vi "ReportVelocityState.vi"(1 "Destination":T3={"Subsystem Id"=90, "Node Id"=1, "Component Id"=1}, 2 "PresenceVector":u16=2 format="%b", 3 "VelocityState":T1, 4 "Source":T3={"Subsystem Id"=3, "Node Id"=1, "Component Id"=1}) -> (0 "Encoded JAUS Message":string)   [LabVIEW 2009]
uses:
  Support Files/Address.ctl
  Support Files/VelocityState.ctl
  Support Files/TimeRec.ctl
panel:
  in  "Command Code":string="D\u0004"
  # "Only Velocity X, Yaw Rate and Time Stamp need to be supplied"
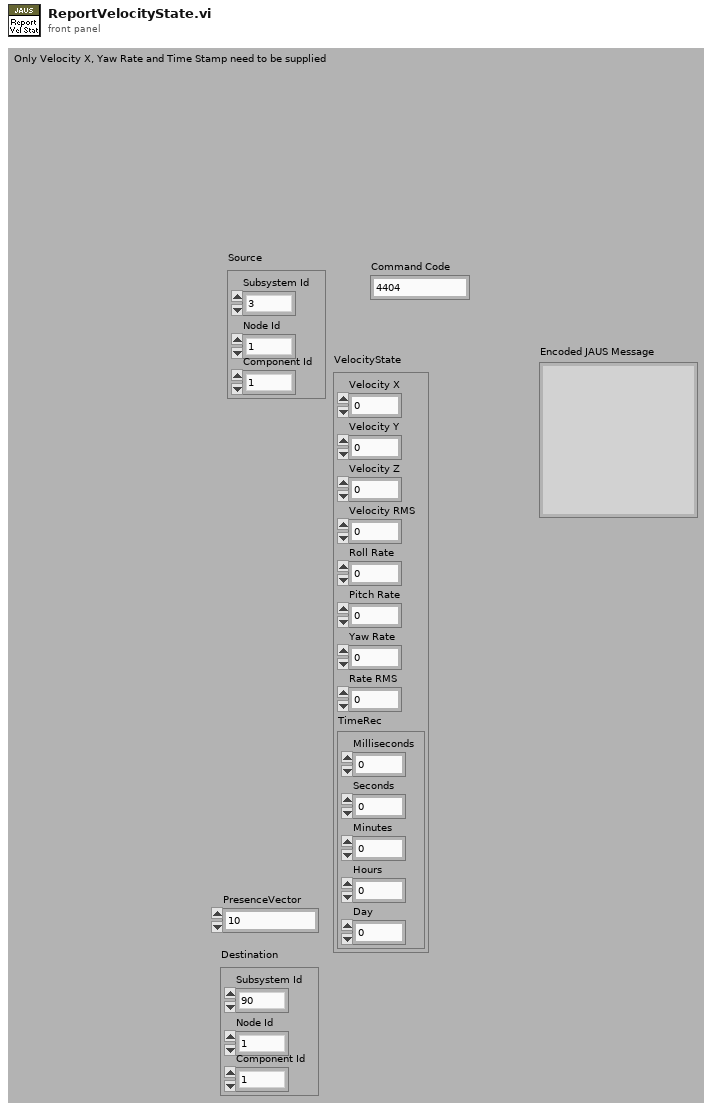
[diagram p1: front panel]
types:
  T1 = typedef "VelocityState.ctl" = cluster{"Velocity X":dbl, "Velocity Y":dbl, "Velocity Z":dbl, "Velocity RMS":dbl, "Roll Rate":dbl, "Pitch Rate":dbl, "Yaw Rate":dbl, "Rate RMS":dbl, "TimeRec":T2}
  T2 = typedef "TimeRec.ctl" = cluster{"Milliseconds":u32, "Seconds":u32, "Minutes":u32, "Hours":u32, "Day":u32}
  T3 = typedef "Address.ctl" = cluster{"Subsystem Id":u16, "Node Id":u8, "Component Id":u8}
  T4 = cluster{"unsigned byte array[0]":u8, "unsigned byte array[1]":u8}
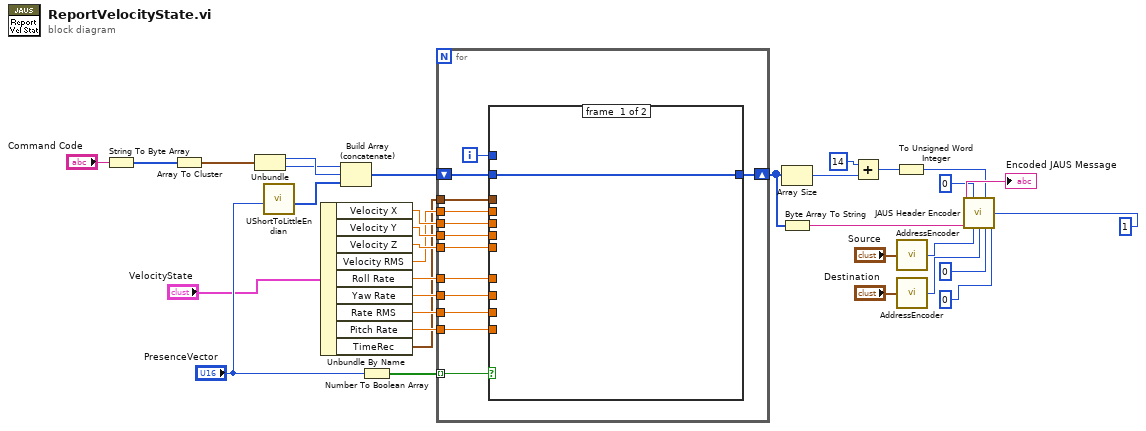
[diagram p0: block diagram]
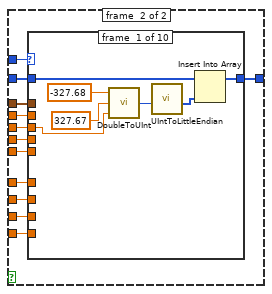
[diagram p2: hidden frame]
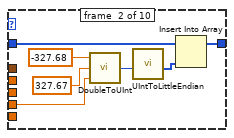
[diagram p3: hidden frame]
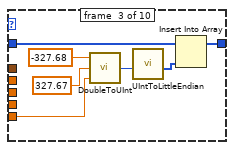
[diagram p4: hidden frame]
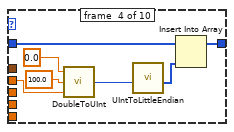
[diagram p5: hidden frame]
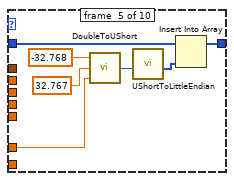
[diagram p6: hidden frame]
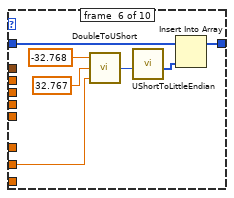
[diagram p7: hidden frame]
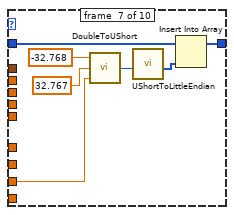
[diagram p8: hidden frame]
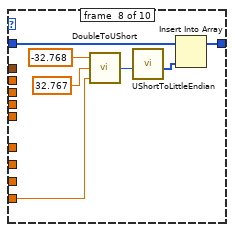
[diagram p9: hidden frame]
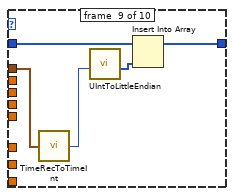
[diagram p10: hidden frame]
diagram:
  n1 = String To Byte Array(string="Command Code") -> (unsigned byte array=w17:u8[])
  n2 = Array To Cluster(array=w17) -> (cluster=w16:T4)
  n3 = Unbundle(w16) -> ("unsigned byte array[0]"=w15:u8, "unsigned byte array[1]"=w14:u8)
  n4 = call "UShortToLittleEndian.vi"("Number"="PresenceVector") -> ("byte array"=w22:u8[])  [unwired: 10 in]
  n5 = Unbundle By Name("VelocityState") -> ("Velocity X"=w13:dbl, "Velocity Y"=w12:dbl, "Velocity Z"=w11:dbl, "Velocity RMS"=w10:dbl, "Roll Rate"=w9:dbl, "Yaw Rate"=w8:dbl, "Rate RMS"=w7:dbl, "Pitch Rate"=w6:dbl, "TimeRec"=w5:T2)
  n6 = Build Array (concatenate)(w14, w15, w22) -> (w20:u8[])
  n7 = Number To Boolean Array(number="PresenceVector") -> (Boolean array=w25:bool[])
  n8 = for {
    tunnel: w25 -> [w47] mode=indexing
    tunnel: w13 -> [w45]
    tunnel: w12 -> [w44]
    tunnel: w11 -> [w43]
    tunnel: w10 -> [w42]
    tunnel: w9 -> [w41]
    tunnel: w8 -> [w40]
    tunnel: w7 -> [w39]
    tunnel: w6 -> [w38]
    tunnel: w5 -> [w37]
    shift-right: [w35] -> w19
    shift-left: w20 -> [w36]
    i -> [w46]
    n9 = case shown="True" w47 {
      tunnel: w46 -> [_ w60]
      tunnel: w45 -> [_ w59]
      tunnel: w44 -> [_ w58]
      tunnel: w43 -> [_ w57]
      tunnel: w42 -> [_ w56]
      tunnel: w41 -> [_ w55]
      tunnel: w40 -> [_ w54]
      tunnel: w39 -> [_ w53]
      tunnel: w38 -> [_ w52]
      tunnel: w37 -> [_ w51]
      tunnel: w36 -> [w48 w50]
      tunnel: [w48 w49] -> w35
      frame #0 {
      }
      frame #1 {
        n10 = case shown="8" w60 {
          tunnel: w59 -> [w63 _ _ _ _ _ _ _ _ _]
          tunnel: w58 -> [_ w70 _ _ _ _ _ _ _ _]
          tunnel: w57 -> [_ _ w77 _ _ _ _ _ _ _]
          tunnel: w56 -> [_ _ _ w84 _ _ _ _ _ _]
          tunnel: w55 -> [_ _ _ _ w91 _ _ _ _ _]
          tunnel: w54 -> [_ _ _ _ _ w98 _ _ _ _]
          tunnel: w53 -> [_ _ _ _ _ _ w105 _ _ _]
          tunnel: w52 -> [_ _ _ _ _ _ _ w112 _ _]
          tunnel: w51 -> [_ _ _ _ _ _ _ _ w120 _]
          tunnel: w50 -> [w62 w69 w76 w83 w90 w97 w104 w111 w118 w122]
          tunnel: [w61 w68 w75 w82 w89 w96 w103 w110 w117 w122] -> w49
          frame #0 {
            n11 = call "DoubleToUInt.vi"("Value"=w63, "Max"=327.67, "Min"=-327.68) -> ("scaled Integer"=w65:u32)
            n12 = call "UIntToLittleEndian.vi"("Number"=w65) -> ("byte array"=w64:u8[])  [unwired: 10 in]
            n13 = Insert Into Array(array=w62, new element=w64) -> (w61:u8[])  [unwired: 1 in]
          }
          frame #1 {
            n14 = call "DoubleToUInt.vi"("Value"=w70, "Max"=327.67, "Min"=-327.68) -> ("scaled Integer"=w72:u32)
            n15 = call "UIntToLittleEndian.vi"("Number"=w72) -> ("byte array"=w71:u8[])  [unwired: 10 in]
            n16 = Insert Into Array(array=w69, new element=w71) -> (w68:u8[])  [unwired: 1 in]
          }
          frame #2 {
            n17 = call "DoubleToUInt.vi"("Value"=w77, "Max"=327.67, "Min"=-327.68) -> ("scaled Integer"=w79:u32)
            n18 = call "UIntToLittleEndian.vi"("Number"=w79) -> ("byte array"=w78:u8[])  [unwired: 10 in]
            n19 = Insert Into Array(array=w76, new element=w78) -> (w75:u8[])  [unwired: 1 in]
          }
          frame #3 {
            n20 = call "DoubleToUInt.vi"("Value"=w84, "Max"=100.0, "Min"=0.0) -> ("scaled Integer"=w86:u32)
            n21 = call "UIntToLittleEndian.vi"("Number"=w86) -> ("byte array"=w85:u8[])  [unwired: 10 in]
            n22 = Insert Into Array(array=w83, new element=w85) -> (w82:u8[])  [unwired: 1 in]
          }
          frame #4 {
            n23 = call "DoubleToUShort.vi"("Value"=w91, "Max"=32.767, "Min"=-32.768) -> ("scaled Integer"=w93:u16)
            n24 = call "UShortToLittleEndian.vi"("Number"=w93) -> ("byte array"=w92:u8[])  [unwired: 10 in]
            n25 = Insert Into Array(array=w90, new element=w92) -> (w89:u8[])  [unwired: 1 in]
          }
          frame #5 {
            n26 = call "DoubleToUShort.vi"("Value"=w98, "Max"=32.767, "Min"=-32.768) -> ("scaled Integer"=w100:u16)
            n27 = call "UShortToLittleEndian.vi"("Number"=w100) -> ("byte array"=w99:u8[])  [unwired: 10 in]
            n28 = Insert Into Array(array=w97, new element=w99) -> (w96:u8[])  [unwired: 1 in]
          }
          frame #6 {
            n29 = call "DoubleToUShort.vi"("Value"=w105, "Max"=32.767, "Min"=-32.768) -> ("scaled Integer"=w107:u16)
            n30 = call "UShortToLittleEndian.vi"("Number"=w107) -> ("byte array"=w106:u8[])  [unwired: 10 in]
            n31 = Insert Into Array(array=w104, new element=w106) -> (w103:u8[])  [unwired: 1 in]
          }
          frame #7 {
            n32 = call "DoubleToUShort.vi"("Value"=w112, "Max"=32.767, "Min"=-32.768) -> ("scaled Integer"=w114:u16)
            n33 = call "UShortToLittleEndian.vi"("Number"=w114) -> ("byte array"=w113:u8[])  [unwired: 10 in]
            n34 = Insert Into Array(array=w111, new element=w113) -> (w110:u8[])  [unwired: 1 in]
          }
          frame #8 {
            n35 = call "TimeRecToTimeInt.vi"("TimeRec"=w120) -> ("timeInt"=w119:u32)
            n36 = call "UIntToLittleEndian.vi"("Number"=w119) -> ("byte array"=w121:u8[])  [unwired: 10 in]
            n37 = Insert Into Array(array=w118, new element=w121) -> (w117:u8[])  [unwired: 1 in]
          }
          frame #9 {
          }
        }
      }
    }
  }
  n38 = Array Size(array=w19) -> (size(s)=w2:i32)
  n39 = Byte Array To String(unsigned byte array=w19) -> (string=w24:string)
  n40 = Add(x=14, y=w2) -> (x+y=w1:i32)
  n41 = To Unsigned Word Integer(number=w1) -> (unsigned 16bit integer=w21:u16)
  n42 = call "AddressEncoder.vi"("Address Cluster"="Source") -> ("Address"=w33:u32)
  n43 = call "AddressEncoder.vi"("Address Cluster"="Destination") -> ("Address"=w32:u32)
  n44 = call "JAUS Header Encoder.vi"("Message Type (0-5)"=u8 0, "Data Size (8-23)"=w21, "Priority(40-41)"=u8 1, "Payload"=w24, "Source ID (80-95)"=w33, "Destination ID (48-79)"=w32, "Data Flags (46-47)"=u8 0, "Ack/Nak (44-45)"=u8 0) -> ("Encoded JAUS Message"=→"Encoded JAUS Message":string)  [unwired: 7 in]
